vi "SVT Third-octave Analysis (1 Ch).vi"(0 "scaled signal [EU]":waveform(dbl)={"t0"=timestamp(0 s since 1904-01-01), "dt"=1.953125e-05, "Y"=[]}, 1 "restart averaging (F)":bool, 2 "reset filter (F)":bool, 5 "frequency range":T8={"low band"=enum."20 Hz", "high band"=enum."20000 Hz"}, 9 "dB On (T)":bool=TRUE, 11 "error in (no error)":errorcluster, 12 "averaging type":T6(ring), 13 "exp avg settings":T1={" mode"=enum."Fast", "time constant [ms]"=125.0} {"time constant [ms]" format="%.2f"}, 14 "equal confidence level [dB]":dbl=125.0 format="%.2f") -> (3 "filter settled":bool, 4 "octave spectrum":T7 {"band power" format="%.2f"; "nominal frequencies [Hz]" format="%.2f"}, 6 "unit label":string, 8 "total band power":dbl format="%.2f", 10 "octave info":T2={"standard"=enum."ANSI S1.11", "bandwidth"=enum."1 octave", "low band"=0, "high band"=0, "weighting filter"=0, "dB reference"=0.0, "dB On"=FALSE, "unit label"="", "channel name"="", "description"="", "engineering units"=1, "custom label"="", "spectrum type"=enum."magnitude", "spectral density"=FALSE, "filters settled"=FALSE} {"engineering units" items=["custom..."=0, "V"=1, "A"=21, "C"=30, "pC"=31, "s"=32, "-"=29, "Pa"=2, "N"=20, "g"=3, "m/s^2"=4, "m/s"=5, "m"=6, "mm/s"=12, "mm"=13, "micron/s"=14, "micron"=15, "in/s^2"=7, "in/s"=8, "in"=9, "mil/s"=10, "mil"=11, "rad/s^2"=16, "rad/s"=17, "rad"=18, "deg/s^2"=26, "deg/s"=27, "deg"=28, "RPM"=22, "cycle/s^2"=23, "Hz"=24, "cycle"=25, "strain"=19]; "dB reference" format="%.2e"; "weighting filter" items=["Linear", "A-weighting", "B-weighting", "C-weighting", "ITU-R 468-4", "Dolby", "CCITT", "C-message", "Wb", "Wc", "Wd", "We", "Wf", "Wh", "Wj", "Wk", "Wm", "AES17 20 kHz lowpass", "AES17 40 kHz lowpass", "AES17 20 kHz highpass", "AES17 40 kHz highpass"]}, 15 "error out":errorcluster)   [LabVIEW 2017, in "SoundVib_Octave.lvlib"]
doc: "LabVIEW no longer supports this VI. The SVT Third-octave Analysis VI is available for compatibility with previous versions of the LabVIEW Sound and Vibration Toolkit. This version of the SVT Third-octave Analysis VI performs a third-octave analysis on <B>scaled signal [EU]</B> in accordance with the IEC 1260 standard. This standard has been superseded by the new IEC 61260 standard. If you want to ensure compliance with the latter standard, use the SVT Third-octave Analysis VI, located on the Octave Analysis palette instead. \n\nYou can use this polymorphic VI to perform third-octave analysis on a single channel or on N channels. The data type you wire to the <B>scaled signal [EU]</B> input determines the polymorphic instance to use."
uses:
  <vilib>/addons/Sound and Vibration/svt_Octave/SoundVib_Octave.lvlib
  <vilib>/addons/Sound and Vibration/svt_Octave/subVIs/sv_Octave Info.ctl
  <vilib>/addons/_NISVFA/_Shared subVIs/Controls/svc_Octave Standard.ctl
  <vilib>/addons/_NISVFA/_Shared subVIs/Controls/svc_Weighting Filter Text Ring.ctl
  <vilib>/addons/_NISVFA/_Shared subVIs/Controls/svc_Engineering Units Text Ring.ctl
  <vilib>/addons/Sound and Vibration/svt_Octave_2014 standard/SoundVib_Octave_2014 standard.lvlib
panel:
  out "# samples to settle":u64
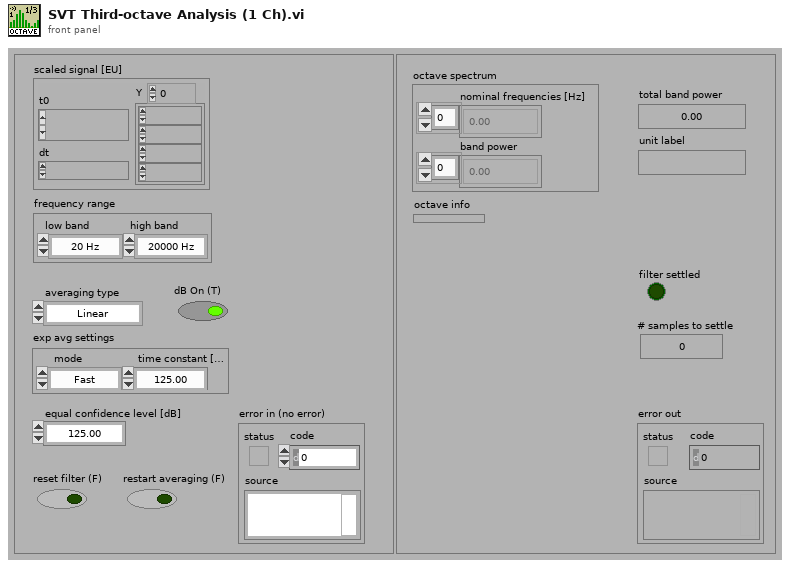
[diagram p1: front panel]
types:
  T1 = cluster{" mode":enum16{"Slow", "Fast", "Impulse", "Custom"}, "time constant [ms]":dbl}
  T2 = typedef "SoundVib_Octave.lvlib/sv_Octave Info.ctl" = cluster{"standard":T3, "bandwidth":enum16{"1 octave", "1/3 octave", "1/6 octave", "1/12 octave", "1/24 octave"}, "low band":i32, "high band":i32, "weighting filter":T4, "dB reference":dbl, "dB On":bool, "unit label":string, "channel name":string, "description":string, "engineering units":T5, "custom label":string, "spectrum type":enum16{"power", "magnitude"}, "spectral density":bool, "filters settled":bool}
  T3 = typedef "svc_Octave Standard.ctl" = enum16{"ANSI S1.11", "IEC 61260"}
  T4 = typedef "svc_Weighting Filter Text Ring.ctl" = u16
  T5 = typedef "svc_Engineering Units Text Ring.ctl" = u16
  T6 = enum16{"Linear", "Exponential", "Equal confidence", "Peak"}
  T7 = cluster{"nominal frequencies [Hz]":dbl[], "band power":dbl[]}
  T8 = cluster{"low band":enum16{"20 Hz", "25 Hz", "31.5 Hz", "40 Hz", "50 Hz", "63 Hz", "80 Hz", "100 Hz", "125 Hz", "160 Hz", "200 Hz", "250 Hz", "315 Hz", "400 Hz", "500 Hz", "630 Hz", "800 Hz", "1000 Hz", "1250 Hz", "1600 Hz", "2000 Hz", "2500 Hz", "3150 Hz", "4000 Hz", "5000 Hz", "6300 Hz", "8000 Hz", "10000 Hz", "12500 Hz", "16000 Hz", "20000 Hz"}, "high band":enum16{"20 Hz", "25 Hz", "31.5 Hz", "40 Hz", "50 Hz", "63 Hz", "80 Hz", "100 Hz", "125 Hz", "160 Hz", "200 Hz", "250 Hz", "315 Hz", "400 Hz", "500 Hz", "630 Hz", "800 Hz", "1000 Hz", "1250 Hz", "1600 Hz", "2000 Hz", "2500 Hz", "3150 Hz", "4000 Hz", "5000 Hz", "6300 Hz", "8000 Hz", "10000 Hz", "12500 Hz", "16000 Hz", "20000 Hz"}}
  T9 = cluster{"standard":T3, "bandwidth":enum16{"1 octave", "1/3 octave", "1/6 octave", "1/12 octave", "1/24 octave"}}
  T10 = cluster{"nominal frequencies [Hz]":dbl[], "band power [EU^2 rms]":dbl[]}
  T11 = typedef "svc_Octave Info.ctl" = cluster{"standard":T3, "bandwidth":enum16{"1 octave", "1/3 octave", "1/6 octave", "1/12 octave", "1/24 octave"}, "low band":i32, "high band":i32, "weighting filter":T4, "dB reference":dbl, "dB On":bool, "unit label":string, "channel name":string, "description":string, "engineering units":T5, "custom label":string, "spectrum type":enum16{"power", "magnitude"}, "spectral density":bool, "filters settled":bool}
  T12 = cluster{"nominal frequencies [Hz]":dbl[], "band power [dB EU]":dbl[]}
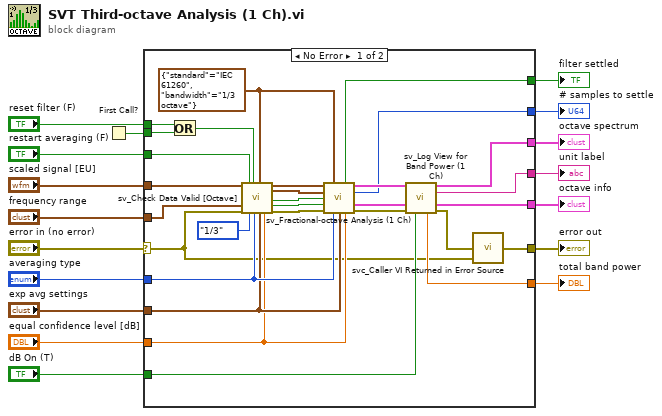
[diagram p0: block diagram]
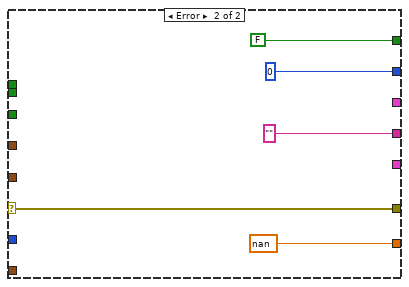
[diagram p2: hidden frame]
diagram:
  n1 = First Call?() -> (First Call?: T/F=w16:bool)
  n2 = case shown="No Error" "error in (no error)" {
    selector: "error in (no error)" -> [w18 w51]
    tunnel: "reset filter (F)" -> [w43 _]
    tunnel: w16 -> [w42 _]
    tunnel: [w41 nan ("total band power [dB EU]")] -> w15
    tunnel: [w22 FALSE ("settled?")] -> w14
    tunnel: "restart averaging (F)" -> [w40 _]
    tunnel: "averaging type" -> [w38 _]
    tunnel: "dB On (T)" -> [w37 _]
    tunnel: "frequency range" -> [w35 _]
    tunnel: "exp avg settings" -> [w34 _]
    tunnel: "equal confidence level [dB]" -> [w20 _]
    tunnel: [w27 w51] -> w7
    tunnel: [w30 _] -> w6
    tunnel: [w29 "" ("unit label")] -> w5
    tunnel: [w28 _] -> w4
    tunnel: "scaled signal [EU]" -> [w26 _]
    tunnel: [w19 u64 0 ("# samples to settle")] -> w1
    frame No Error {
      w24 = T9 {"standard"=enum."IEC 61260", "bandwidth"=enum."1/3 octave"} ("1/n Octave settings")
      n3 = Or(x=w43, y=w42) -> (x .or. y?=w25:bool)
      n4 = call <vilib>:"sv_Check Data Valid [Octave].vi"("scaled signal [EU]"=w26, "frequency range (1/3)"=w35, "error in (no error)"=w18, "restart averaging (F)"=w40, "bandwidth"=enum16{"1/1", "1/3", "1/n"}."1/3", "reset filter (F)"=w25, "averaging type"=w38, "1/n octave settings"=w24, "exp avg settings"=w34, "equal confidence level [dB]"=w20) -> ("dup scaled signal [EU]"=w45:waveform(dbl), "band number"=w33:cluster{"low band":i32, "high band":i32}, "Restart averaging"=w39:bool, "Reset Filter"=w21:bool, "error out"=w46:errorcluster)  [unwired: 5 in]
      n5 = call <vilib>:"sv_Fractional-octave Analysis (1 Ch).vi"("scaled signal [EU]"=w45, "1/n Octave settings"=w24, "band number"=w33, "restart averaging (F)"=w39, "reset filter (F)"=w21, "error in (no error)"=w46, "averaging type"=w38, "exp avg settings"=w34, "equal confidence level [dB]"=w20) -> ("settled?"=w22:bool, "octave spectrum"=w36:T10, "# samples to settle"=w19:u64, "octave info"=w31:T11, "error out"=w44:errorcluster)  [unwired: 2 in]
      n6 = call <vilib>:"sv_Log View for Band Power (1 Ch).vi"("octave spectrum"=w36, "octave info"=w31, "error in (no error)"=w44, "dB On (T)"=w37) -> ("octave spectrum"=w30:T12, "unit label"=w29:string, "octave info"=w28:T11, "total band power [dB EU]"=w41:dbl, "error out"=w32:errorcluster)  [unwired: 7 in]
      n7 = call <vilib>:"svc_Caller VI Returned in Error Source.vi"("warning input to caller"=w18, "error in (no error)"=w32) -> ("error out"=w27:errorcluster)  [unwired: 3 in]
    }
    frame Error {
    }
  }
  "filter settled" <- w14
  "unit label" <- w5
  "total band power" <- w15
  "error out" <- w7
  "octave spectrum" <- w6
  "octave info" <- w4
  "# samples to settle" <- w1
